vi "Update Meter.vi"(8 "error in (no error)":errorcluster, 10 "Update Meter":dbl, 11 "Business Logic in":refnum<class "Business Logic.lvclass">) -> (0 "error out":errorcluster, 3 "Business Logic out":refnum<class "Business Logic.lvclass">)   [LabVIEW 2020, in "Business Logic.lvlib" / "Business Logic.lvclass"]
uses:
  Business Logic.lvclass
  Business Logic.lvclass/Business Logic.ctl
  Indicators Messages/Update Meter Msg/Update Meter Msg.lvclass
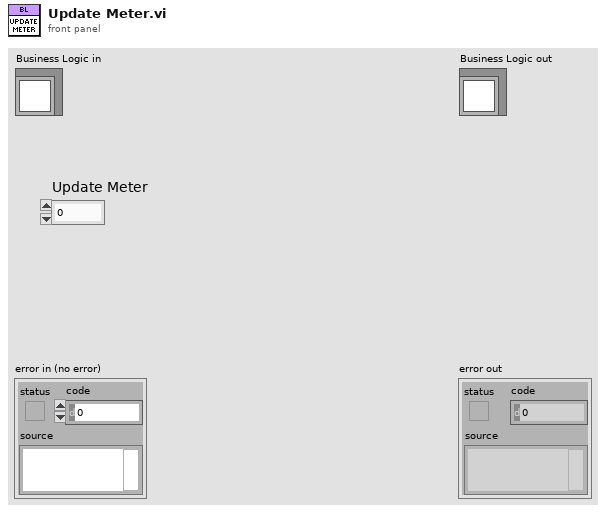
[diagram p1: front panel]
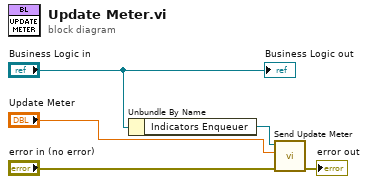
[diagram p0: block diagram]
diagram:
  n1 = Unbundle By Name("Business Logic in") -> ("Indicators Enqueuer"=w1:refnum<class "Message Enqueuer.lvclass">)
  n2 = call "Send Update Meter.vi"("error in (no error)"="error in (no error)", "Meter"="Update Meter", "Message Enqueuer"=w1) -> ("error out"=→"error out":errorcluster)  [unwired: 7 in, 1 out]
  "Business Logic out" <- "Business Logic in"
